vi "Comm Down.vi"(8 "error in (no error)":errorcluster, 11 "DAQ Actor in":refnum<class "DAQ Actor.lvclass">) -> (0 "error out":errorcluster, 3 "DAQ Actor out":refnum<class "DAQ Actor.lvclass">)   [LabVIEW 2018, in "Data Acquisition.lvlib" / "DAQ Actor.lvclass"]
uses:
  DAQ Actor.lvclass
  C:/Program Files (x86)/National Instruments/LabVIEW 2018/vi.lib/ActorFramework/Actor/Actor.lvclass
  <vilib>/ActorFramework/Actor/Actor.lvclass/Actor.ctl
  <vilib>/ActorFramework/Message Enqueuer/Message Enqueuer.lvclass/Message Enqueuer.ctl
  DAQ Actor.lvclass/DAQ Actor.ctl
  <vilib>/ActorFramework/Message Enqueuer/Init from Existing Queue.vi
  <vilib>/ActorFramework/Message Enqueuer/Enqueue.vi
  DAQ Actor Messages/Comm Down Msg/Comm Down Msg.lvclass
  C:/Program Files (x86)/National Instruments/LabVIEW 2018/vi.lib/ActorFramework/Message/Message.lvclass
  <vilib>/ActorFramework/Message Priority Queue/Priority Enqueue.vi
  <vilib>/ActorFramework/Message Enqueuer/Message Enqueuer.lvclass
  <vilib>/ActorFramework/Actor/Actor.lvclass
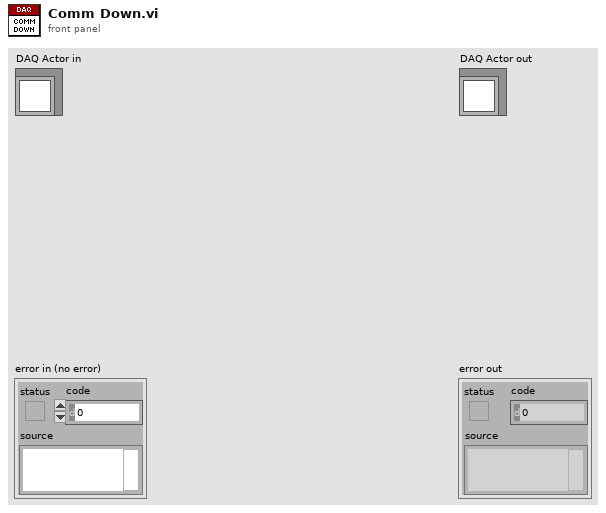
[diagram p1: front panel]
types:
  T1 = typedef "Telnet Session.ctl" = refnum<k1>
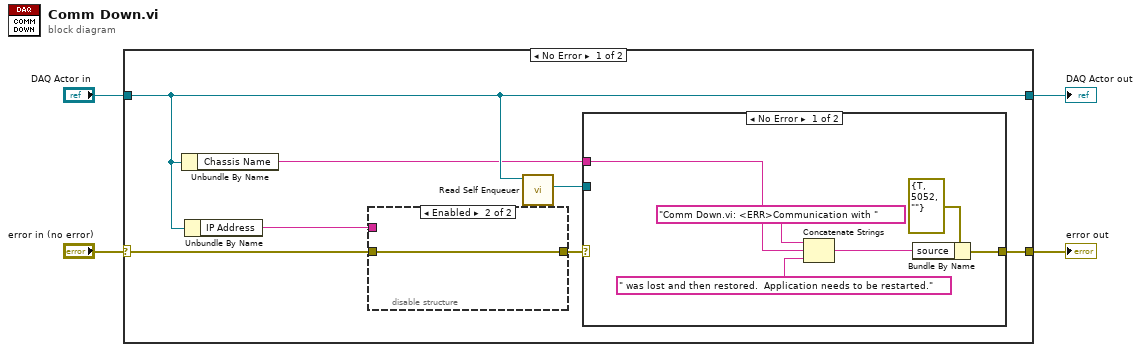
[diagram p0: block diagram]
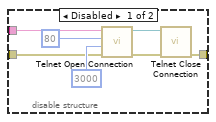
[diagram p2: hidden frame]
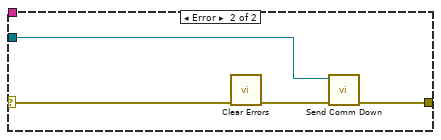
[diagram p3: hidden frame]
diagram:
  n1 = case shown="No Error" "error in (no error)" {
    selector: "error in (no error)" -> [w6 w31]
    tunnel: [w10 w31] -> w3
    tunnel: [w8 w30] -> w1
    tunnel: "DAQ Actor in" -> [w8 w30]
    frame No Error {
      n2 = Unbundle By Name(w8) -> ("Chassis Name"=w5:string)
      n3 = Unbundle By Name(w8) -> ("IP Address"=w7:string)
      n4 = disable-structure shown="Enabled" {
        disable-tunnel: [w16 w19] -> w11
        disable-tunnel: w7 -> [w13 _]
        disable-tunnel: w6 -> [w12 w19]
        frame Disabled {
          n5 = call <vilib>:"Telnet Open Connection.vi"("error in (no error)"=w12, "timeout ms (60000)"=3000, "remote port (23)"=u16 80, "address"=w13) -> ("error out"=w15:errorcluster, "telnet connection"=w17:T1)  [unwired: 6 in]
          n6 = call <vilib>:"Telnet Close Connection.vi"("error in (no error)"=w15, "telnet connection"=w17) -> ("error out"=w16:errorcluster)  [unwired: 8 in, 1 out]
        }
        frame Enabled {
        }
      }
      n7 = call <vilib>:"Read Self Enqueuer.vi"("Actor"=w8) -> ("Self Enqueuer"=w9:refnum<class "Message Enqueuer.lvclass">)  [unwired: 10 in]
      n8 = case shown="No Error" w11 {
        selector: w11 -> [_ w29]
        tunnel: [w21 w27] -> w10
        tunnel: w5 -> [w20 _]
        tunnel: w9 -> [_ w26]
        frame No Error {
          n9 = Concatenate Strings("Comm Down.vi: <ERR>Communication with ", w20, " was lost and then restored.  Application needs to be restarted.") -> (w22:string)
          n10 = Bundle By Name(cluster=errorcluster {"status"=TRUE, "code"=5052, "source"=""} ("error IO"), "source"=w22) -> (w21:errorcluster)
        }
        frame Error {
          n11 = call <vilib>:"Clear Errors.vi"("error in (no error)"=w29) -> ("error out"=w28:errorcluster)  [unwired: 5 in, 1 out]
          n12 = call "Send Comm Down.vi"("error in (no error)"=w28, "Message Enqueuer"=w26) -> ("error out"=w27:errorcluster)  [unwired: 8 in, 1 out]
        }
      }
    }
    frame Error {
    }
  }
  "error out" <- w3
  "DAQ Actor out" <- w1
